vi "InitADS1115.vi"(8 "error in (no error)":errorcluster, 9 "Grove Connector":enum16{"I2C0", "I2C1"}(ring), 10 "Address":u8, 11 "VISA Refnum in":refnum<visa-resource-name>) -> (0 "error out":errorcluster, 2 "Bus":u8, 3 "VISA Refnum out":refnum<visa-resource-name>)   [LabVIEW 2024]
uses:
  Driver/Public/Digital Pull Direction.ctl
  Driver/CTIPicoVISA.lvlib
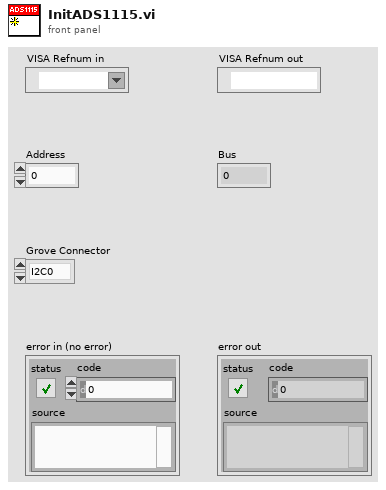
[diagram p1: front panel]
types:
  T1 = typedef "CTIPicoVISA.lvlib/Digital Pull Direction.ctl" = enum16{"None", "Up", "Down", "Both"}
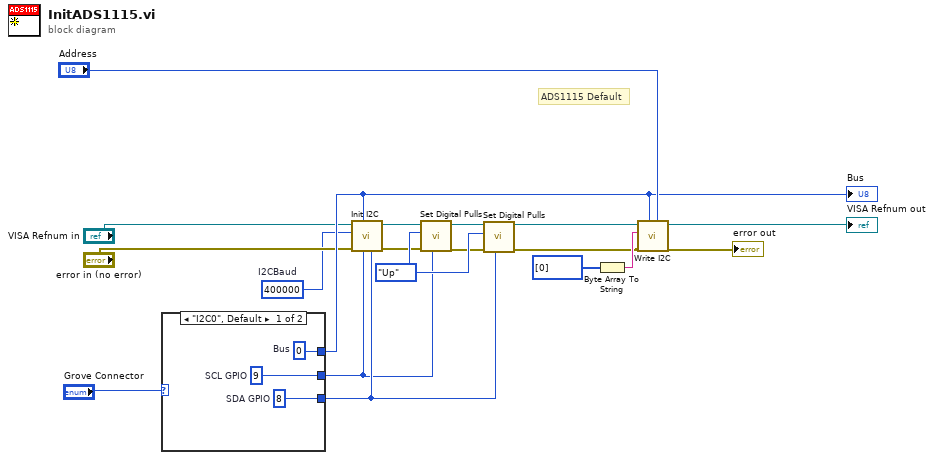
[diagram p0: block diagram]
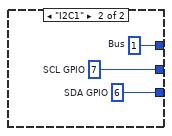
[diagram p2: hidden frame]
diagram:
  w8 = Digital_Pull_Direction."Up" ("Pull")
  w1 = u32 400000  # I2CBaud
  # "ADS1115 Default"
  n1 = case shown="\"I2C0\", Default" "Grove Connector" {
    tunnel: [w22 w25] -> w7
    tunnel: [w21 w24] -> w9
    tunnel: [w20 w23] -> w15
    frame "I2C0", Default {
      w20 = u8 0  # Bus
      w21 = 8  # SDA GPIO
      w22 = 9  # SCL GPIO
    }
    frame "I2C1" {
      w23 = u8 1  # Bus
      w24 = 6  # SDA GPIO
      w25 = 7  # SCL GPIO
    }
  }
  "Bus" <- w15
  n2 = call "Init I2C.vi"("SDA GPIO"=w9, "SCL GPIO"=w7, "Bus"=w15, "error in (no error)"="error in (no error)", "Baud"=w1, "VISA resource name in"="VISA Refnum in") -> ("error out"=w4:errorcluster, "VISA resource name"=w3:refnum<visa-resource-name>)  [unwired: 4 in]
  n3 = call "Set Digital Pulls.vi"("GPIO"=w7, "error in (no error)"=w4, "Pull"=w8, "VISA resource name in"=w3) -> ("error out"=w6:errorcluster, "VISA resource name"=w5:refnum<visa-resource-name>)  [unwired: 6 in]
  n4 = call "Set Digital Pulls.vi"("GPIO"=w9, "error in (no error)"=w6, "Pull"=w8, "VISA resource name in"=w5) -> ("error out"=w14:errorcluster, "VISA resource name"=w13:refnum<visa-resource-name>)  [unwired: 6 in]
  n5 = Byte Array To String(unsigned byte array=u8[] [0]) -> (string=w17:string)
  n6 = call "Write I2C.vi"("Address"="Address", "Bus"=w15, "error in (no error)"=w14, "Data"=w17, "VISA resource name in"=w13) -> ("error out"=→"error out":errorcluster, "VISA resource name"=→"VISA Refnum out":refnum<visa-resource-name>)  [unwired: 5 in]
